vi "一天一张EXCEL.vi"(8 "error in (no error)":errorcluster caption="错误输入（无错误）", 10 "其余文件夹名称":string[](array[string])) -> (0 "error out":errorcluster caption="错误输出", 1 "EXCEL文件存在？":bool, 2 "dup path":path caption="路径副本")   [LabVIEW 2014]
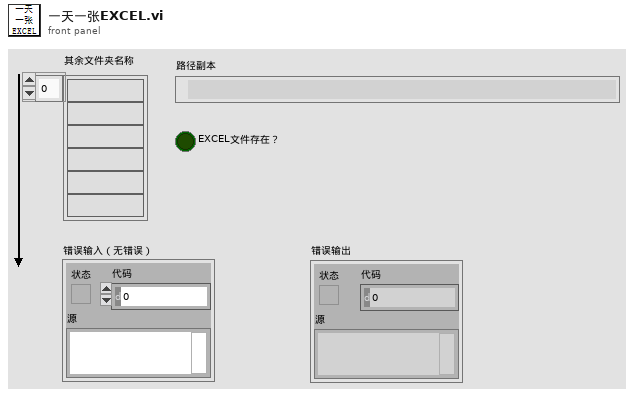
[diagram p1: front panel]
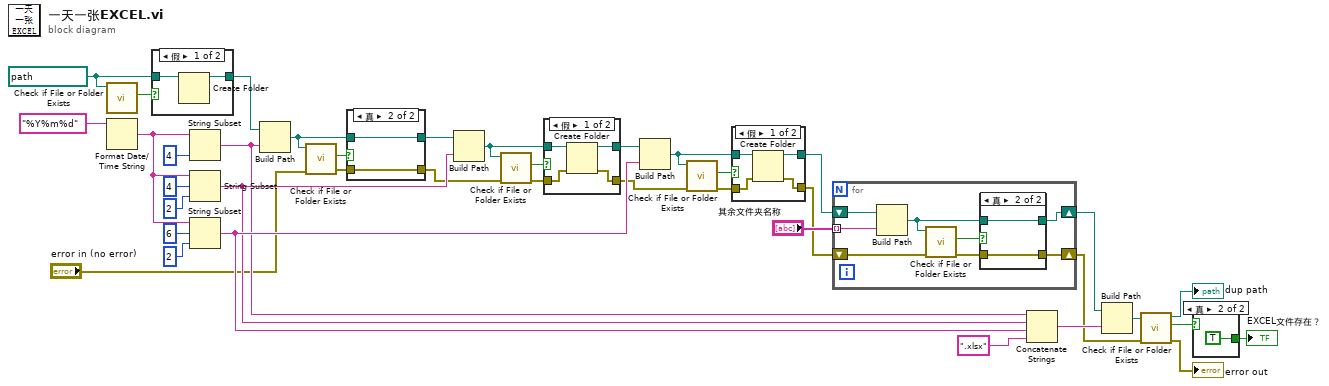
[diagram p0: block diagram]
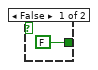
[diagram p2: hidden frame]
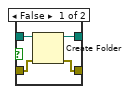
[diagram p3: hidden frame]
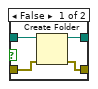
[diagram p6: hidden frame]
diagram:
  w27 = path "D:/数据保存" ("path")
  n1 = call <vilib>:"Check if File or Folder Exists.vi"("path"=w27) -> ("file or folder exists?"=w26:bool)  [unwired: 8 in, 2 out]
  n2 = Format Date/Time String(time format string (%c)="%Y%m%d" ("时间格式字符串(%c)")) -> (date/time string=w23:string)  [unwired: 2 in]
  n3 = case shown="假" w26 {
    tunnel: w27 -> [w41 w42]
    tunnel: [w40 w42] -> w28
    frame False {
      n4 = Create Folder(path (use dialog)=w41) -> (created path=w40:path)  [unwired: 2 in, 2 out]
    }
    frame True {
    }
  }
  n5 = String Subset(string=w23, length (rest)=4 ("长度（剩余）")) -> (substring=w37:string)  [unwired: 1 in]
  n6 = String Subset(string=w23, offset (0)=4 ("偏移量(0)"), length (rest)=2 ("长度（剩余）")) -> (substring=w38:string)
  n7 = String Subset(string=w23, offset (0)=6 ("偏移量(0)"), length (rest)=2 ("长度（剩余）")) -> (substring=w39:string)
  n8 = Build Path(base path=w28, name or relative path=w37) -> (appended path=w30:path)
  n9 = call <vilib>:"Check if File or Folder Exists.vi"("error in (no error)"="error in (no error)", "path"=w30) -> ("error out"=w8:errorcluster, "file or folder exists?"=w29:bool)  [unwired: 7 in, 1 out]
  n10 = case shown="真" w29 {
    tunnel: w30 -> [w46 w48]
    tunnel: [w45 w48] -> w32
    tunnel: w8 -> [w44 w47]
    tunnel: [w43 w47] -> w7
    frame False {
      n11 = Create Folder(path (use dialog)=w46, error in=w44) -> (created path=w45:path, error out=w43:errorcluster)  [unwired: 1 in, 1 out]
    }
    frame True {
    }
  }
  n12 = Build Path(base path=w32, name or relative path=w38) -> (appended path=w33:path)
  n13 = call <vilib>:"Check if File or Folder Exists.vi"("error in (no error)"=w7, "path"=w33) -> ("error out"=w6:errorcluster, "file or folder exists?"=w31:bool)  [unwired: 7 in, 1 out]
  n14 = case shown="假" w31 {
    tunnel: w33 -> [w52 w54]
    tunnel: [w51 w54] -> w36
    tunnel: w6 -> [w50 w53]
    tunnel: [w49 w53] -> w5
    frame False {
      n15 = Create Folder(path (use dialog)=w52, error in=w50) -> (created path=w51:path, error out=w49:errorcluster)  [unwired: 1 in, 1 out]
    }
    frame True {
    }
  }
  n16 = Build Path(base path=w36, name or relative path=w39) -> (appended path=w34:path)
  n17 = call <vilib>:"Check if File or Folder Exists.vi"("error in (no error)"=w5, "path"=w34) -> ("error out"=w4:errorcluster, "file or folder exists?"=w35:bool)  [unwired: 7 in, 1 out]
  n18 = case shown="假" w35 {
    tunnel: w34 -> [w58 w60]
    tunnel: [w57 w60] -> w17
    tunnel: w4 -> [w56 w59]
    tunnel: [w55 w59] -> w3
    frame False {
      n19 = Create Folder(path (use dialog)=w58, error in=w56) -> (created path=w57:path, error out=w55:errorcluster)  [unwired: 1 in, 1 out]
    }
    frame True {
    }
  }
  n20 = for {
    tunnel: "其余文件夹名称" -> [w65] mode=indexing
    shift-right: [w64] -> w13
    shift-left: w17 -> [w66]
    shift-right: [w61] -> w2
    shift-left: w3 -> [w63]
    n21 = Build Path(base path=w66, name or relative path=w65) -> (appended path=w68:path)
    n22 = call <vilib>:"Check if File or Folder Exists.vi"("error in (no error)"=w63, "path"=w68) -> ("error out"=w62:errorcluster, "file or folder exists?"=w67:bool)  [unwired: 7 in, 1 out]
    n23 = case shown="真" w67 {
      tunnel: w68 -> [w72 w74]
      tunnel: [w71 w74] -> w64
      tunnel: w62 -> [w70 w73]
      tunnel: [w69 w73] -> w61
      frame False {
        n24 = Create Folder(path (use dialog)=w72, error in=w70) -> (created path=w71:path, error out=w69:errorcluster)  [unwired: 1 in, 1 out]
      }
      frame True {
      }
    }
  }
  n25 = Concatenate Strings(w37, w38, w39, ".xlsx" ("字符串")) -> (w16:string)
  n26 = Build Path(base path=w13, name or relative path=w16) -> (appended path=w15:path)
  n27 = call <vilib>:"Check if File or Folder Exists.vi"("error in (no error)"=w2, "path"=w15) -> ("error out"=→"error out":errorcluster, "file or folder exists?"=w12:bool, "dup path"=→"dup path":path)  [unwired: 7 in]
  n28 = case shown="真" w12 {
    tunnel: [FALSE TRUE] -> w10
    frame False {
    }
    frame True {
    }
  }
  "EXCEL文件存在？" <- w10
